vi "5RobotsFactorPass.vi"(0 "Utilities in":refnum<class "Utilities.lvclass">, 1 "ID":dbl, 5 "Game in":refnum<class "Game.lvclass">, 7 "reference":refnum<class "Enemy.lvclass">, 9 "Root":dbl=1.0, 11 "error in (no error)":errorcluster, 12 "Pass?":bool, 13 "Enemy?":bool, 14 "dest_kick":dbl[][](array[numeric])) -> (3 "Debug":dbl[][](array[numeric]), 4 "Utilities out":refnum<class "Utilities.lvclass">, 6 "Id":i32[](array[numeric]), 10 "FactorPass":dbl[](array[numeric]), 15 "error out":errorcluster)   [LabVIEW 2021, in "Utilities.lvclass"]
uses:
  Utilities.lvclass
  Game_class/Game.lvclass
  Enemy_class/Enemy.lvclass
  D:/RoboIme/horie/SSL_AI/Team_class/Team.lvclass
  Game_class/Game.lvclass/Game.ctl
  Team_class/Team.lvclass/Team.ctl
  Object_class/Object.lvclass/Object.ctl
  Robot_class/roles.ctl
  Robot_class/Robot.lvclass/Robot.ctl
  Team_class/OffensivePlay.ctl
  Referee_class/Referee.lvclass/Referee.ctl
  Object_class/Read position(x,y).vi
  Team_class/Read RobotRef.vi
  Robot_class/Read id.vi
  Object_class/Read x.vi
  Object_class/Read y.vi
  Referee_class/Read enemy_goalie_id.vi
  Referee_class/Read our_goalie_id.vi
  Game_class/Read OffensiveTeam.vi
  Game_class/Read BallRef.vi
  Game_class/Read FieldRef.vi
  Game_class/Read EnemyRef.vi
  Game_class/Read Referee.vi
  Ally_class/Ally.lvclass
  Robot_class/Robot.lvclass
  D:/RoboIme/horie/SSL_AI/Object_class/Object.lvclass
  Ball_class/Ball.lvclass
  Field_class/Field.lvclass
  Referee_class/Referee.lvclass
  Team_class/Team.lvclass
panel:
  in  "y3 2":dbl=0.2
  in  "y4 2":dbl=0.2
  in  "y":dbl=0.2
  in  "y2":dbl=0.22
  in  "y3":dbl=0.35
  in  "y4":dbl=0.16
  in  "y5":dbl=0.07
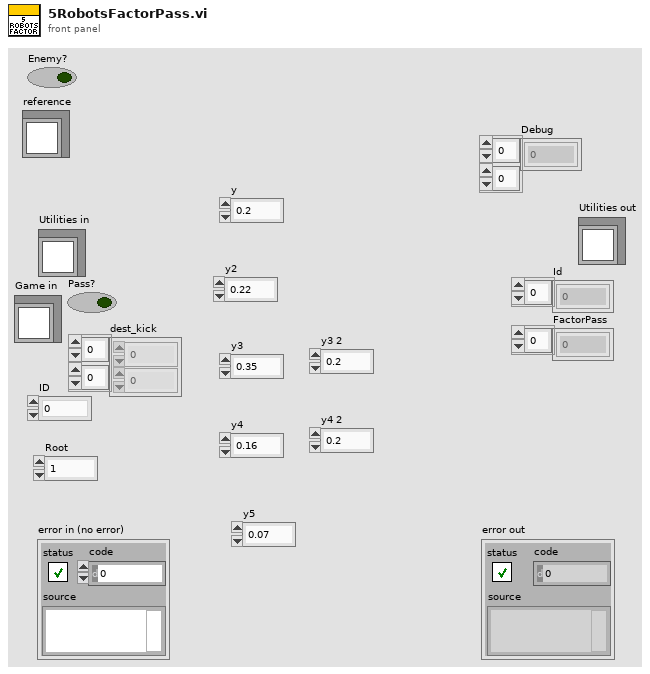
[diagram p1: front panel]
types:
  T1 = typedef "roles.ctl" = enum16{"SimpleBallPlacement", "BallPlacementAllyPasser", "BallPlacementAllyReceiver", "BallPlacementEnemy", "5Robots5th", "PassBestReceiver", "5Robots4th", "5Robots3rd", "5Robots2nd", "5Robots1st", "PassBestRobot", "WaitPass", "ABCThirdKicker", "ABCFirstKicker", "ABCSecondKicker", "Tabler", "TableFinalizer", "PrepareRollToPassRoller", "PrepareRollToPassReceiver", "SimplePassRoll", "SimplePassRollReceiver", "PenaltyDefense", "PreparePassReceiver 2", "PreparePassReceiver 1", "PassObserver", "Timeout", "Goto", "ZigZag", "None", "BallOutOfField", "DefenderArea", "Duelist", "AttackerStop", "FollowAttacker", "KeeperRole", "KickPenalty", "AttackerAimGoal", "AttackerBlock", "Marker", "Halt", "Shoot", "PassKicker", "PassReceiver", "TestRole", "PenaltyAttacker"}
  T2 = typedef "OffensivePlay.ctl" = enum16{"5RobotsPassGamePlay", "5PreparePassGame", "5RobotsKeeperGame", "KeeperPassToStriker", "5RobotsNormalGamePlay", "PrepareKeeperPass", "ACBPass", "ABCPass", "PrepareTriplePass", "TableWithStriker", "TableWith2ndStrikerPlay", "PrepareDoublePass", "PrepareRollToPass", "SimplePass", "PreparePass", "PassToStriker", "BallOutOfField", "PassTo2ndStriker", "StopOffensive", "Prepare Penalty Enemy", "EnemyPossessionAtEnemyField", "EnemyPossesionAtOurField", "TestPlay", "PreparePenaltyAlly", "KickPenaltyAlly", "PrepareKickoffAlly", "PrepareKickoffEnemy", "IndirectEnemy", "DirectEnemy", "PreparePassInGame1", "NormalGame", "DirectKick", "Pass", "Halt", "Timeout", "PassPlay", "PenaltyEnemy"}
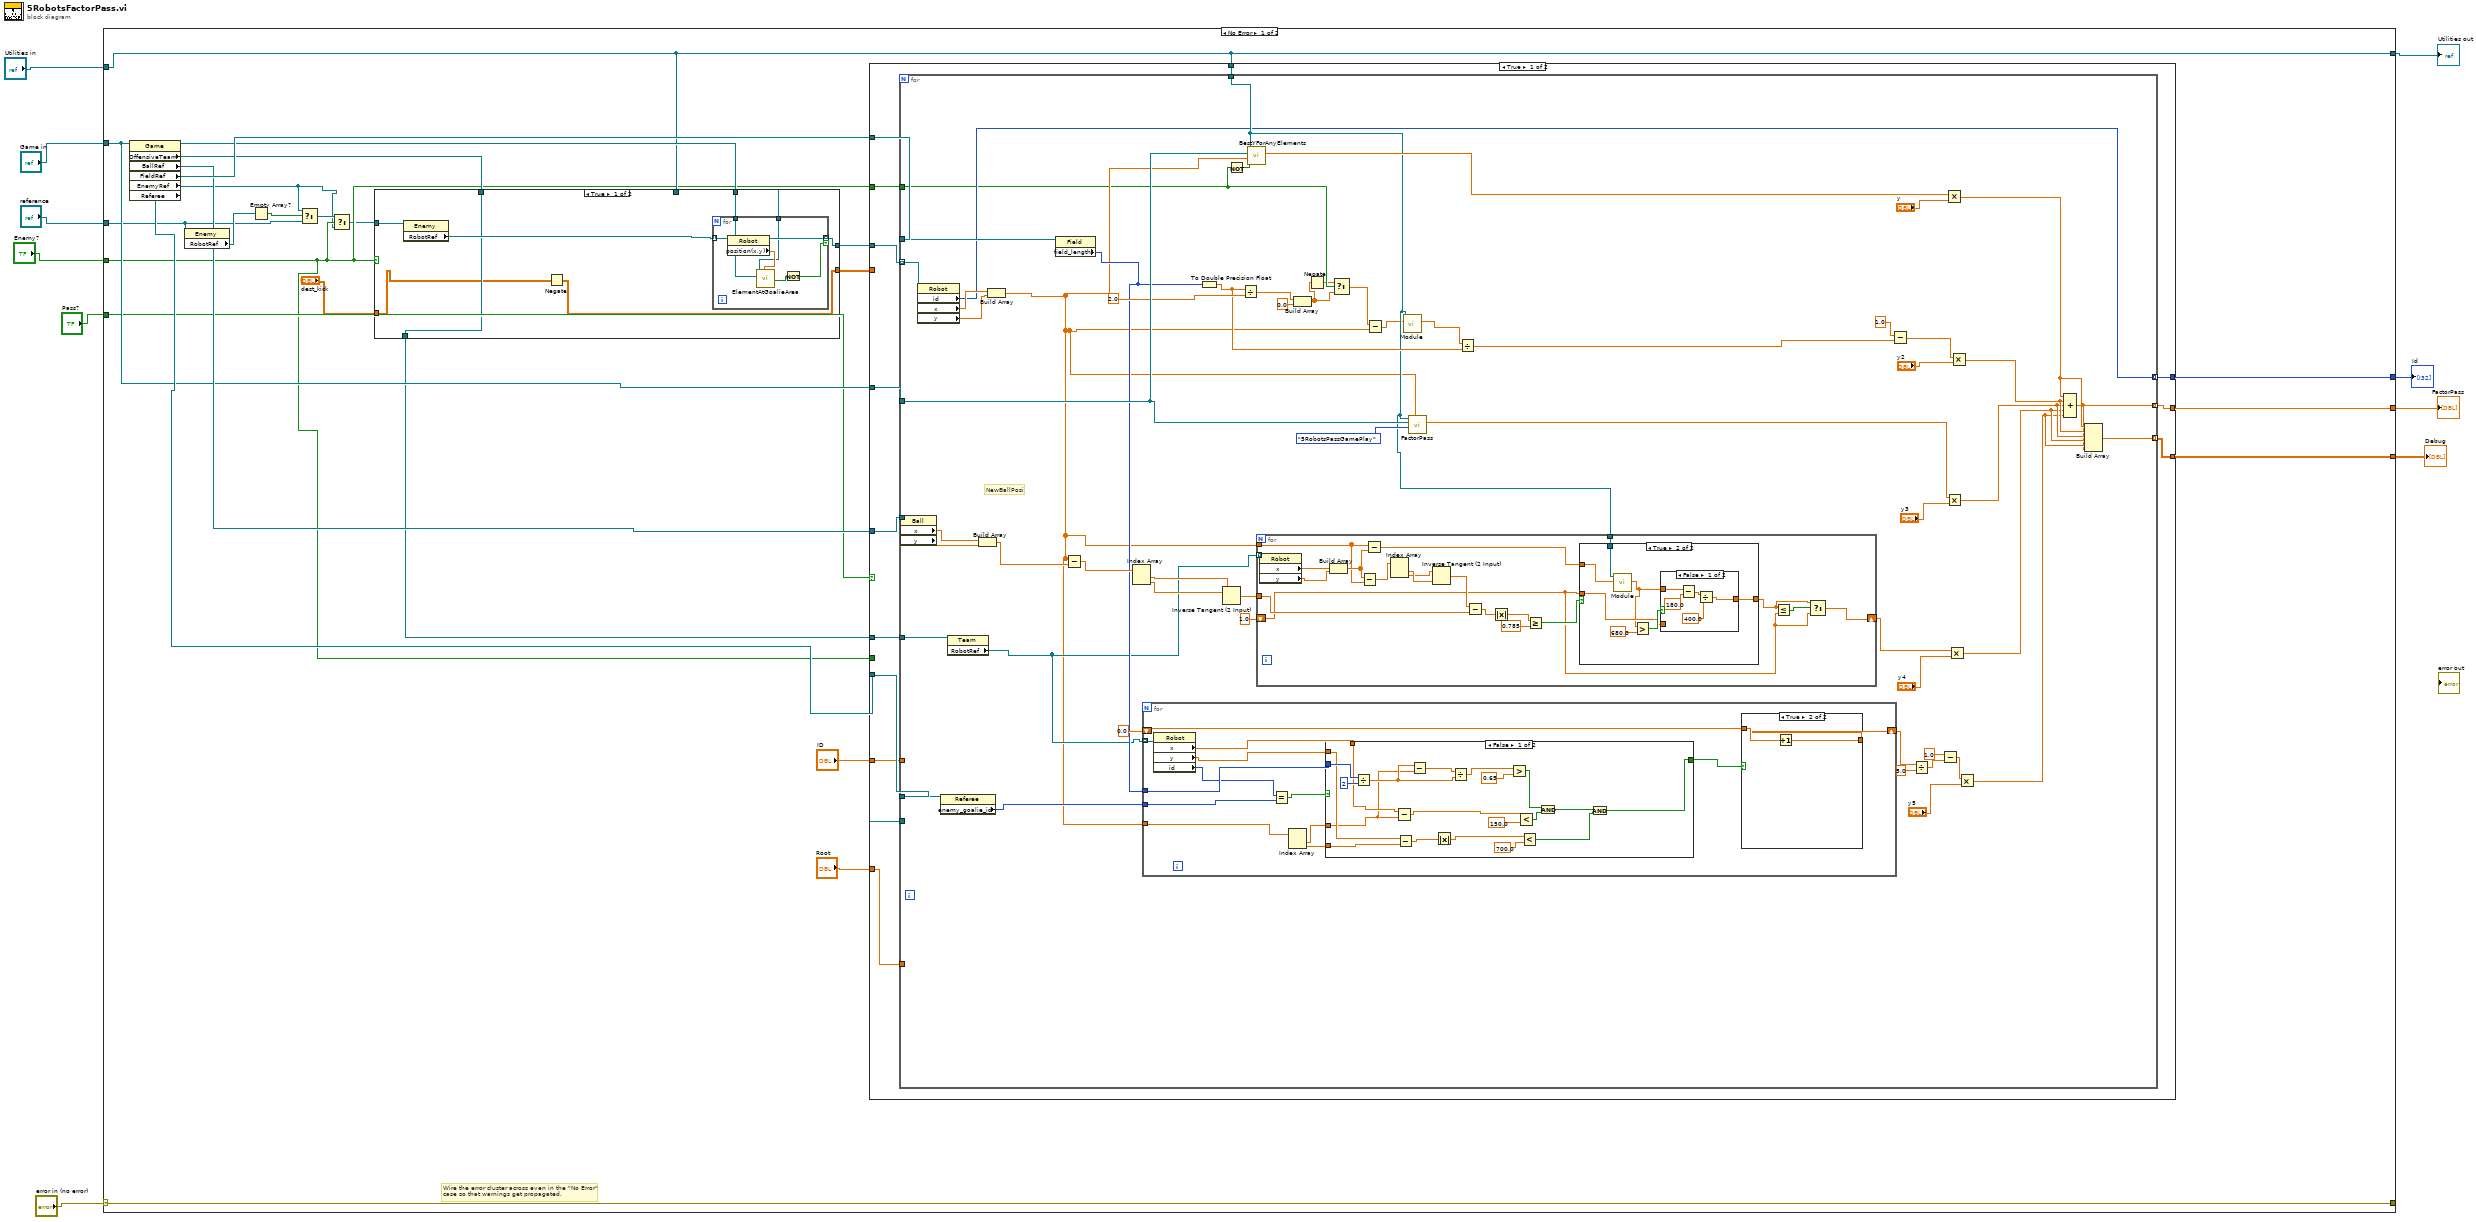
[diagram p0: block diagram]
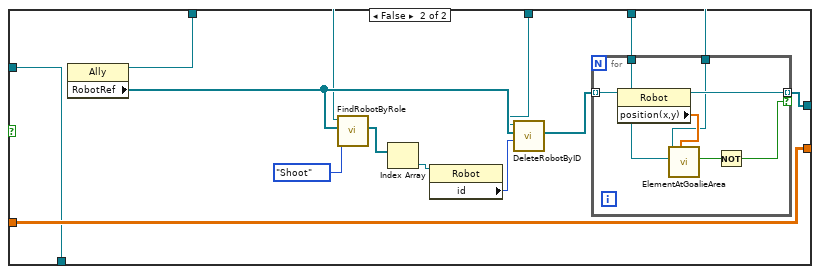
[diagram p2: hidden frame]
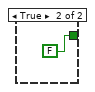
[diagram p3: hidden frame]
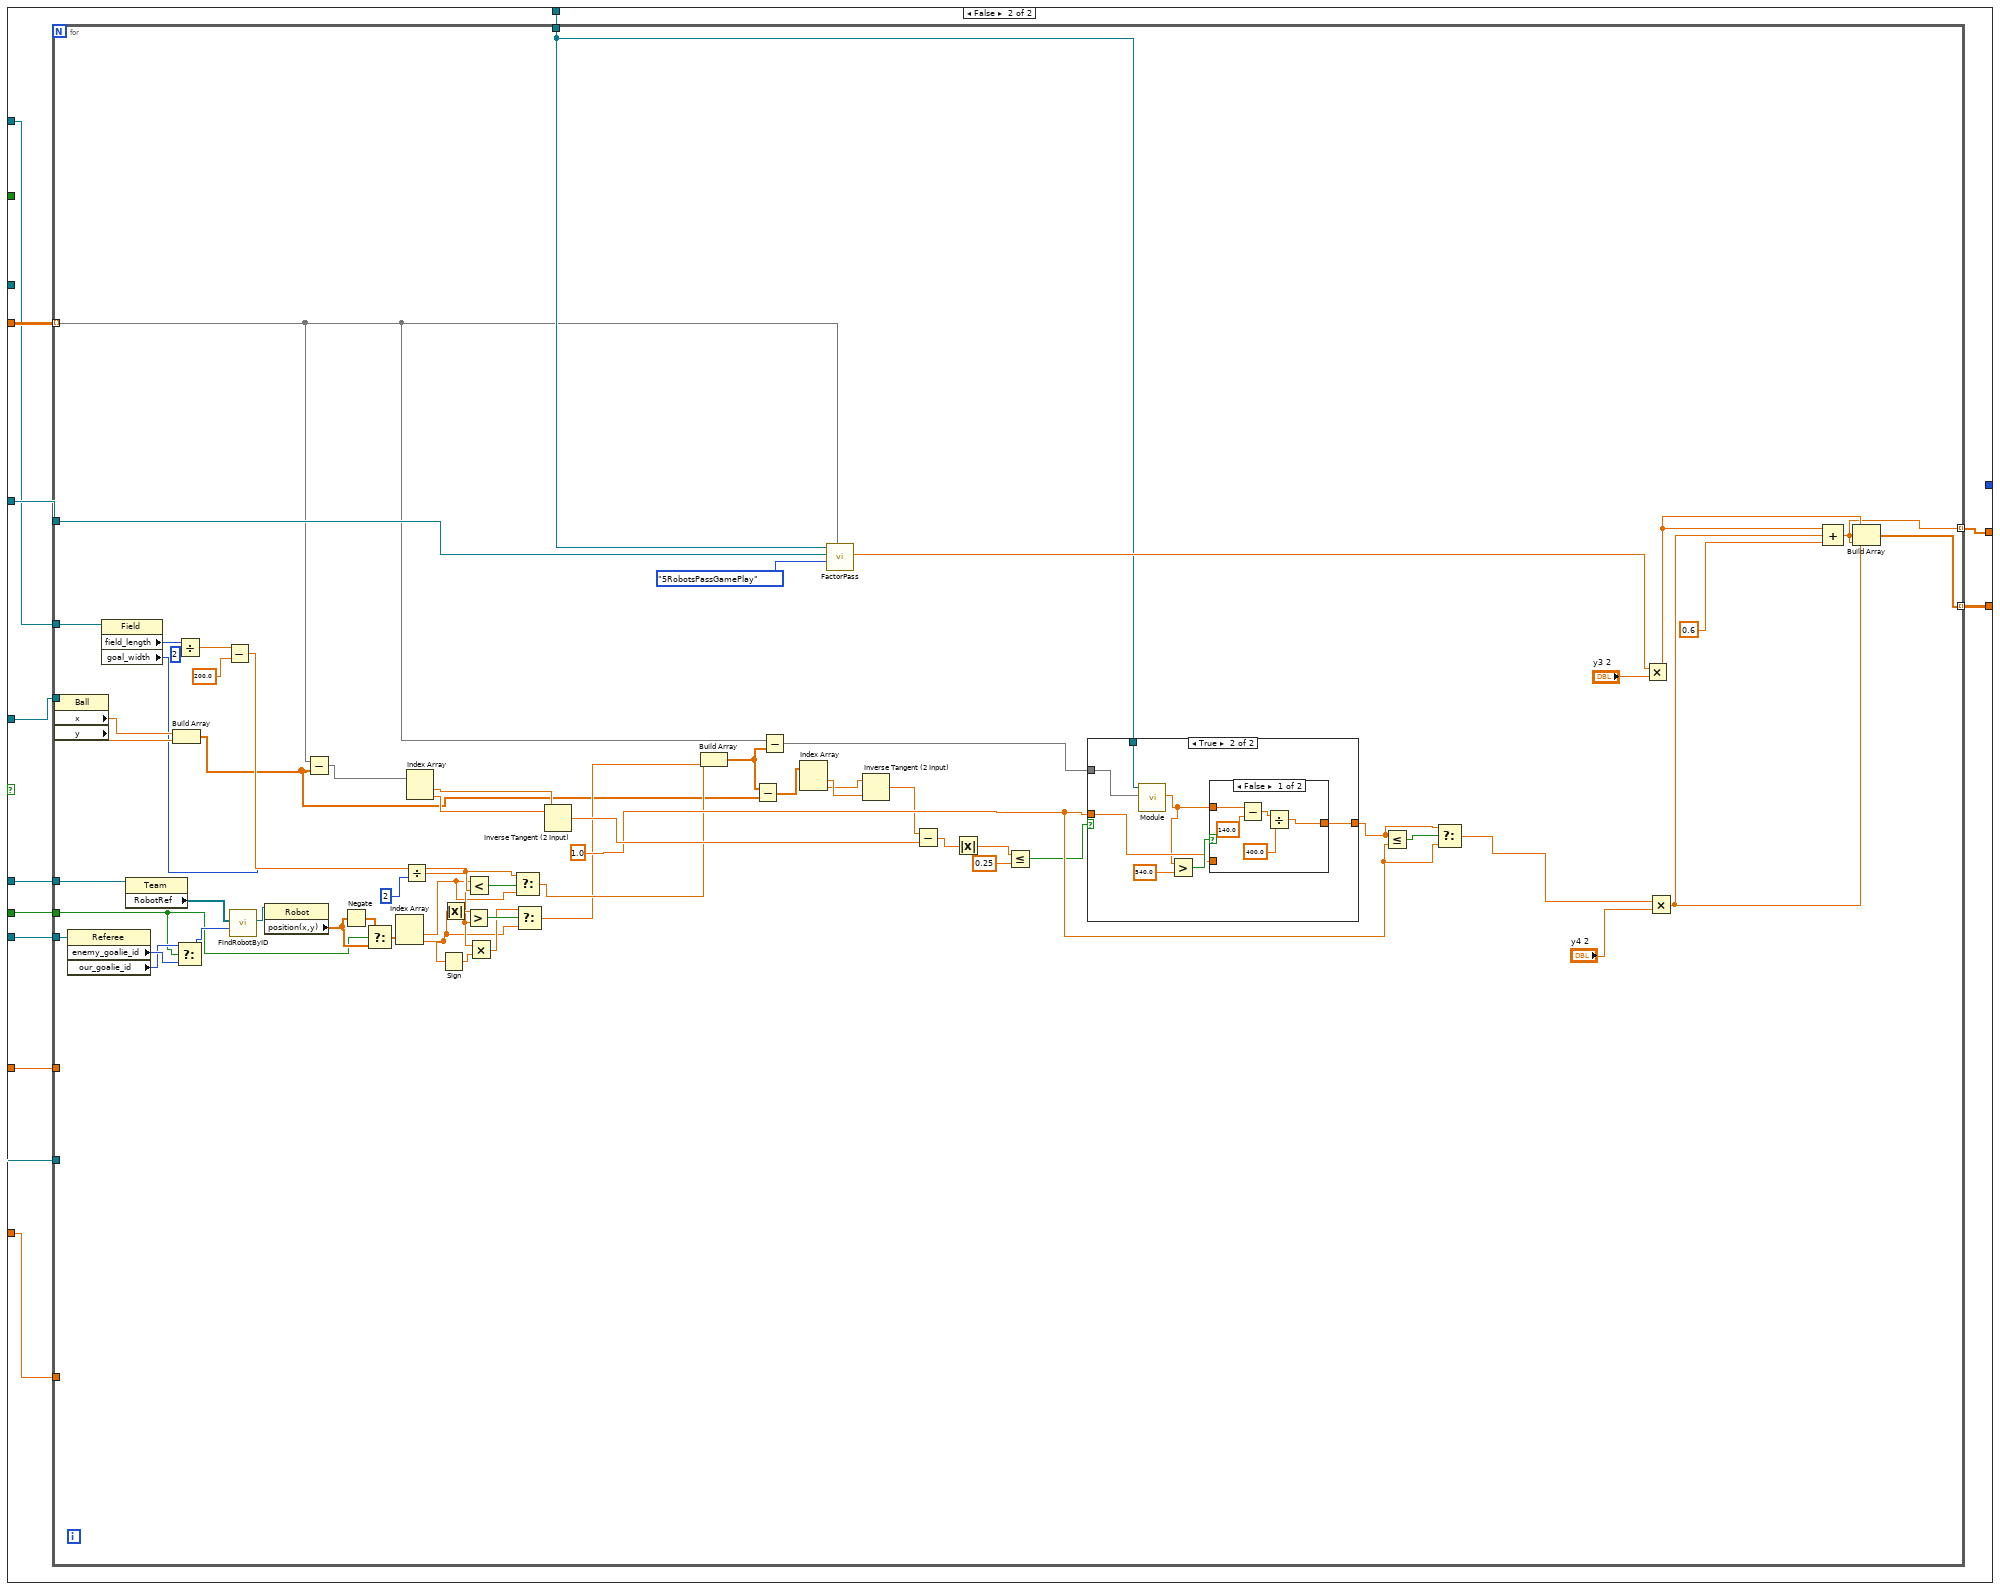
[diagram p7: hidden frame]
diagram:
  n1 = case shown="No Error" "error in (no error)" {
    selector: "error in (no error)" -> [w35 w302]
    tunnel: [w35 w302] -> _
    tunnel: [w31 _] -> w6
    tunnel: "Utilities in" -> [w20 w301]
    tunnel: [w20 w301] -> w10
    tunnel: "Game in" -> [w28 _]
    tunnel: [w29 _] -> w7
    tunnel: "Pass?" -> [w26 _]
    tunnel: [w24 _] -> w3
    tunnel: "Enemy?" -> [w14 _]
    tunnel: "reference" -> [w15 _]
    frame No Error {
      # "Wire the error cluster across even in the \"No Error\"\ncase so that warnings get propagated."
      n2 = property class="Game"(reference=w28) -> (reference out=w22:refnum<class "Game.lvclass">, "OffensiveTeam"=w30:refnum<class "Ally.lvclass">, "BallRef"=w33:refnum<class "Ball.lvclass">, "FieldRef"=w34:refnum<class "Field.lvclass">, "EnemyRef"=w11:refnum<class "Enemy.lvclass">, "Referee"=w32:refnum<class "Referee.lvclass">)  [unwired: 1 in, 1 out]
      n3 = property class="Enemy"(reference=w15) -> ("RobotRef"=w16:refnum<class "Robot.lvclass">[])  [unwired: 1 in, 2 out]
      n4 = Empty Array?(array=w16) -> (empty?=w17:bool)
      n5 = Select(t=w11, s=w17, f=w15) -> (s? t:f=w12:refnum<class "Enemy.lvclass">)
      n6 = Select(t=w12, s=w14, f=w11) -> (s? t:f=w13:refnum<class "Enemy.lvclass">)
      n7 = case shown="True" w14 {
        tunnel: w30 -> [w39 w62]
        tunnel: [w37 w52] -> w25
        tunnel: w22 -> [w43 w56]
        tunnel: [w42 w54] -> w21
        tunnel: w20 -> [w41 w53]
        tunnel: "dest_kick" -> [w38 w52]
        tunnel: [w39 w51] -> w18
        tunnel: w13 -> [w36 w51]
        frame True {
          n8 = property class="Enemy"(reference=w36) -> ("RobotRef"=w40:refnum<class "Robot.lvclass">[])  [unwired: 1 in, 2 out]
          n9 = Negate(x=w38) -> (-x=w37:dbl[][])
          n10 = for {
            tunnel: w43 -> [w50]
            tunnel: w40 -> [w49] mode=indexing
            tunnel: [w47] -> w42 mode=indexing if=w46
            tunnel: w41 -> [w45]
            n11 = property class="Robot"(reference=w49) -> (reference out=w47:refnum<class "Robot.lvclass">, "position(x,y)"=w48:dbl[])  [unwired: 1 in, 1 out]
            n12 = call "ElementAtGoalieArea.vi"("Elemento pos."=w48, "Game"=w50, "Utilities in"=w45) -> ("Element at our goalkeeper area ?"=w44:bool)  [unwired: 4 in, 4 out]
            n13 = Not(x=w44) -> (.not. x?=w46:bool)
          }
        }
        frame False {
          n14 = property class="Ally"(reference=w62) -> ("RobotRef"=w57:refnum<class "Robot.lvclass">[])  [unwired: 1 in, 2 out]
          n15 = call "FindRobotByRole.vi"("role"=roles."Shoot", "RobotRef"=w57, "Utilities in"=w53) -> ("Robots"=w60:refnum<class "Robot.lvclass">[])  [unwired: 6 in, 2 out]
          n16 = Index Array(array=w60) -> (element=w59:refnum<class "Robot.lvclass">)  [unwired: 1 in]
          n17 = property class="Robot"(reference=w59) -> ("id"=w58:i32)  [unwired: 1 in, 2 out]
          n18 = call "DeleteRobotByID.vi"("id"=w58, "RobotRef"=w57, "Utilities in"=w53) -> ("RobotRef out"=w55:refnum<class "Robot.lvclass">[])  [unwired: 6 in, 2 out]
          n19 = for {
            tunnel: w56 -> [w69]
            tunnel: w55 -> [w68] mode=indexing
            tunnel: [w66] -> w54 mode=indexing if=w64
            tunnel: w53 -> [w63]
            n20 = property class="Robot"(reference=w68) -> (reference out=w66:refnum<class "Robot.lvclass">, "position(x,y)"=w67:dbl[])  [unwired: 1 in, 1 out]
            n21 = call "ElementAtGoalieArea.vi"("Elemento pos."=w67, "Game"=w69, "Utilities in"=w63) -> ("Element at any goalkeeper area ?"=w65:bool)  [unwired: 4 in, 4 out]
            n22 = Not(x=w65) -> (.not. x?=w64:bool)
          }
        }
      }
      n23 = case shown="True" w26 {
        tunnel: w34 -> [w82 w213]
        tunnel: w33 -> [w81 w223]
        tunnel: w18 -> [w80 w222]
        tunnel: w32 -> [w79 w214]
        tunnel: [w78 w221] -> w31
        tunnel: w20 -> [w77 w220]
        tunnel: w21 -> [w76 _]
        tunnel: [w75 _] -> w29
        tunnel: w28 -> [w74 w219]
        tunnel: "ID" -> [w73 w218]
        tunnel: "Root" -> [w72 w215]
        tunnel: w25 -> [_ w217]
        tunnel: [w71 w216] -> w24
        tunnel: w14 -> [w70 _]
        tunnel: w14 -> [_ w212]
        frame True {
          n24 = for {
            tunnel: w82 -> [w140]
            tunnel: w81 -> [w139]
            tunnel: w80 -> [w138]
            tunnel: w79 -> [w137]
            tunnel: [w90] -> w78 mode=indexing
            tunnel: w74 -> [w136]
            tunnel: w77 -> [w100]
            tunnel: w76 -> [w104] mode=indexing
            tunnel: [w99] -> w75 mode=indexing
            tunnel: w72 -> [_]
            tunnel: w74 -> [_]
            tunnel: w73 -> [_]
            tunnel: [w93] -> w71 mode=indexing
            tunnel: w70 -> [w86]
            # "NewBallPosi"
            n25 = property class="Ball"(reference=w139) -> ("x"=w124:dbl, "y"=w123:dbl)  [unwired: 1 in, 2 out]
            n26 = property class="Robot"(reference=w104) -> ("id"=w99:i32, "x"=w103:dbl, "y"=w102:dbl)  [unwired: 1 in, 2 out]
            n27 = property class="Referee"(reference=w137) -> ("enemy_goalie_id"=w106:i32)  [unwired: 1 in, 2 out]
            n28 = property class="Team"(reference=w138) -> ("RobotRef"=w107:refnum<class "Robot.lvclass">[])  [unwired: 1 in, 2 out]
            n29 = Build Array(w124, w123) -> (w89:dbl[])
            n30 = Build Array(w103, w102) -> (w87:dbl[])
            n31 = property class="Field"(reference=w140) -> ("field_length"=w109:i32)  [unwired: 1 in, 2 out]
            n32 = Subtract(x=w87, y=w89) -> (x-y=w122:dbl[])
            n33 = Index Array(array=w122) -> (element #1=w120:dbl, element #2=w121:dbl)  [unwired: 2 in]
            n34 = for {
              tunnel: w87 -> [w147]
              shift-right: [w152] -> w115
              shift-left: 0.0 -> [w153]
              tunnel: w106 -> [w151]
              tunnel: w109 -> [w148]
              tunnel: w107 -> [w144] mode=indexing
              n35 = property class="Robot"(reference=w144) -> ("x"=w143:dbl, "y"=w142:dbl, "id"=w141:i32)  [unwired: 1 in, 2 out]
              n36 = Equal?(x=w141, y=w151) -> (x = y?=w150:bool)
              n37 = Index Array(array=w147) -> (element #1=w146:dbl, element #2=w145:dbl)  [unwired: 2 in]
              n38 = case shown="False" w150 {
                tunnel: [w155 FALSE] -> w149
                tunnel: w148 -> [w173 _]
                tunnel: w143 -> [w166 _]
                tunnel: w146 -> [w154 _]
                tunnel: w142 -> [w164 _]
                tunnel: w145 -> [w163 _]
                frame False {
                  n39 = Divide(x=w173, y=u32 2) -> (x/y=w170:dbl)
                  n40 = Subtract(x=w166, y=w154) -> (x-y=w165:dbl)
                  n41 = Subtract(x=w164, y=w163) -> (x-y=w162:dbl)
                  n42 = Subtract(x=w170, y=w154) -> (x-y=w171:dbl)
                  n43 = Absolute Value(x=w162) -> (abs(x)=w161:dbl)
                  n44 = Divide(x=w171, y=w170) -> (x/y=w169:dbl)
                  n45 = Greater?(x=w169, y=0.65) -> (0:w159:bool)
                  n46 = Less?(x=w165, y=150.0) -> (x < y?=w158:bool)
                  n47 = Less?(x=w161, y=700.0) -> (x < y?=w156:bool)
                  n48 = And(x=w159, y=w158) -> (x .and. y?=w157:bool)
                  n49 = And(x=w157, y=w156) -> (x .and. y?=w155:bool)
                }
                frame True {
                }
              }
              n50 = case shown="True" w149 {
                tunnel: w153 -> [w175 w177]
                tunnel: [w175 w176] -> w152
                frame False {
                }
                frame True {
                  n51 = Increment(x=w177) -> (x+1=w176:dbl)
                }
              }
            }
            n52 = To Double Precision Float(number=w109) -> (double precision float=w130:dbl)
            n53 = Inverse Tangent (2 Input)(1:w120, 2:w121) -> (0:w119:dbl)
            n54 = Not(x=w86) -> (.not. x?=w88:bool)
            n55 = Divide(x=w130, y=2.0) -> (x/y=w134:dbl)
            n56 = call "BestYForAnyElements.vi"("inimigos"=w88, "Position to be analyzed"=w87, "Game"=w136, "Utilities in"=w100) -> ("Goal Gap"=w108:dbl)  [unwired: 6 in, 1 out]
            n57 = for {
              tunnel: w119 -> [w192]
              tunnel: w87 -> [w182]
              shift-right: [w184] -> w118
              shift-left: 1.0 ("element") -> [w183]
              tunnel: w107 -> [w181] mode=indexing
              tunnel: w100 -> [w178]
              n58 = property class="Robot"(reference=w181) -> ("x"=w180:dbl, "y"=w179:dbl)  [unwired: 1 in, 2 out]
              n59 = Build Array(w180, w179) -> (w188:dbl[])
              n60 = Subtract(x=w188, y=w182) -> (x-y=w197:dbl[])
              n61 = Subtract(x=w182, y=w188) -> (x-y=w187:dbl[])
              n62 = Index Array(array=w197) -> (element #1=w194:dbl, element #2=w193:dbl)  [unwired: 2 in]
              n63 = Inverse Tangent (2 Input)(1:w194, 2:w193) -> (0:w196:dbl)
              n64 = Subtract(x=w196, y=w192) -> (x-y=w195:dbl)
              n65 = Absolute Value(x=w195) -> (abs(x)=w190:dbl)
              n66 = Greater Or Equal?(x=w190, y=0.785) -> (x >= y?=w189:bool)
              n67 = case shown="True" w189 {
                tunnel: w183 -> [w198 w202]
                tunnel: w187 -> [_ w201]
                tunnel: [w198 w204] -> w185
                tunnel: w178 -> [_ w200]
                frame False {
                }
                frame True {
                  n68 = call "Module.vi"("2D vector"=w201, "Utilities in"=w200) -> ("Modulo"=w199:dbl)  [unwired: 7 in, 2 out]
                  n69 = Greater?(x=w199, y=680.0) -> (0:w203:bool)
                  n70 = case shown="False" w203 {
                    tunnel: w202 -> [_ w211]
                    tunnel: [w210 w211] -> w204
                    tunnel: w199 -> [w206 _]
                    frame False {
                      n71 = Subtract(x=w206, y=180.0) -> (x-y=w208:dbl)
                      n72 = Divide(x=w208, y=400.0) -> (x/y=w210:dbl)
                    }
                    frame True {
                    }
                  }
                }
              }
              n73 = Less Or Equal?(x=w185, y=w183) -> (x <= y?=w186:bool)
              n74 = Select(t=w185, s=w186, f=w183) -> (s? t:f=w184:dbl)
            }
            n75 = Build Array(w134, 0.0 ("element")) -> (w85:dbl[])
            n76 = Negate(x=w85) -> (-x=w84:dbl[])
            n77 = Select(t=w84, s=w86, f=w85) -> (s? t:f=w83:dbl[])
            n78 = Subtract(x=w83, y=w87) -> (x-y=w92:dbl[])
            n79 = call "Module.vi"("2D vector"=w92, "Utilities in"=w100) -> ("Modulo"=w91:dbl)  [unwired: 7 in, 2 out]
            n80 = call-dynamic "FactorPass.vi"("Robot"=w87, "OffensivePlay"=OffensivePlay."5RobotsPassGamePlay", "Game"=w136, "Utilities in"=w100) -> ("Critério de marcação Normalizado"=w105:dbl)  [unwired: 5 in, 2 out]
            n81 = Divide(x=w91, y=w130) -> (x/y=w132:dbl)
            n82 = Subtract(x=1.0, y=w132) -> (x-y=w129:dbl)
            n83 = Divide(x=w115, y=5.0) -> (x/y=w113:dbl)
            n84 = Subtract(x=1.0, y=w113) -> (x-y=w111:dbl)
            n85 = Multiply(x=w108, y="y") -> (x*y=w98:dbl)
            n86 = Multiply(x=w105, y="y3") -> (x*y=w96:dbl)
            n87 = Multiply(x=w118, y="y4") -> (x*y=w95:dbl)
            n88 = Multiply(x=w129, y="y2") -> (x*y=w97:dbl)
            n89 = Multiply(x=w111, y="y5") -> (x*y=w94:dbl)
            n90 = Compound Arithmetic op=ADD(w98, w97, w96, w95, w94) -> (w90:dbl)
            n91 = Build Array(w98, w97, w96, w95, w94, w90) -> (w93:dbl[])
          }
        }
        frame False {
          n92 = for {
            tunnel: w223 -> [w286]
            tunnel: w222 -> [w285]
            tunnel: [w267] -> w221 mode=indexing
            tunnel: w219 -> [w284]
            tunnel: w220 -> [w271]
            tunnel: w215 -> [_]
            tunnel: w219 -> [_]
            tunnel: w218 -> [_]
            tunnel: w217 -> [w224] mode=indexing
            tunnel: [w270] -> w216 mode=indexing
            tunnel: w214 -> [w264]
            tunnel: w213 -> [w263]
            tunnel: w212 -> [w228]
            w274 = 1.0 ("element")
            n93 = property class="Ball"(reference=w286) -> ("x"=w281:dbl, "y"=w280:dbl)  [unwired: 1 in, 2 out]
            n94 = property class="Referee"(reference=w264) -> ("enemy_goalie_id"=w232:i32, "our_goalie_id"=w231:i32)  [unwired: 1 in, 2 out]
            n95 = property class="Field"(reference=w263) -> ("field_length"=w262:i32, "goal_width"=w254:i32)  [unwired: 1 in, 2 out]
            n96 = property class="Team"(reference=w285) -> ("RobotRef"=w265:refnum<class "Robot.lvclass">[])  [unwired: 1 in, 2 out]
            n97 = Build Array(w281, w280) -> (w234:dbl[])
            n98 = Select(t=w231, s=w228, f=w232) -> (s? t:f=w233:i32)
            n99 = Divide(x=w262, y=2) -> (x/y=w260:dbl)
            n100 = Subtract(x=w260, y=200.0) -> (x-y=w256:dbl)
            n101 = call "FindRobotByID.vi"("id"=w233, "RobotRef"=w265) -> ("Robot"=w258:refnum<class "Robot.lvclass">)  [unwired: 6 in, 3 out]
            n102 = property class="Robot"(reference=w258) -> ("position(x,y)"=w230:dbl[])  [unwired: 1 in, 2 out]
            n103 = Subtract(x=w224, y=w234) -> (x-y=w279:dbl[])
            n104 = Negate(x=w230) -> (-x=w229:dbl[])
            n105 = Select(t=w229, s=w228, f=w230) -> (s? t:f=w227:dbl[])
            n106 = Index Array(array=w227) -> (element #1=w226:dbl, element #2=w225:dbl)  [unwired: 2 in]
            n107 = Divide(x=w254, y=2) -> (x/y=w250:dbl)
            n108 = Index Array(array=w279) -> (element #1=w277:dbl, element #2=w278:dbl)  [unwired: 2 in]
            n109 = Sign(1:w225) -> (0:w249:dbl)
            n110 = Absolute Value(x=w225) -> (abs(x)=w252:dbl)
            n111 = Greater?(x=w252, y=w250) -> (0:w251:bool)
            n112 = Less?(x=w226, y=w256) -> (x < y?=w257:bool)
            n113 = Multiply(x=w250, y=w249) -> (x*y=w248:dbl)
            n114 = Select(t=w256, s=w257, f=w226) -> (s? t:f=w255:dbl)
            n115 = Select(t=w248, s=w251, f=w225) -> (s? t:f=w247:dbl)
            n116 = Inverse Tangent (2 Input)(1:w277, 2:w278) -> (0:w276:dbl)
            n117 = Build Array(w255, w247) -> (w235:dbl[])
            n118 = Subtract(x=w235, y=w234) -> (x-y=w246:dbl[])
            n119 = Subtract(x=w224, y=w235) -> (x-y=w238:dbl[])
            n120 = Index Array(array=w246) -> (element #1=w243:dbl, element #2=w242:dbl)  [unwired: 2 in]
            n121 = call-dynamic "FactorPass.vi"("Robot"=w224, "OffensivePlay"=OffensivePlay."5RobotsPassGamePlay", "Game"=w284, "Utilities in"=w271) -> ("Critério de marcação Normalizado"=w273:dbl)  [unwired: 5 in, 2 out]
            n122 = Inverse Tangent (2 Input)(1:w243, 2:w242) -> (0:w245:dbl)
            n123 = Subtract(x=w245, y=w276) -> (x-y=w244:dbl)
            n124 = Absolute Value(x=w244) -> (abs(x)=w240:dbl)
            n125 = Less Or Equal?(x=w240, y=0.25) -> (x <= y?=w239:bool)
            n126 = case shown="True" w239 {
              tunnel: w274 -> [w287 w291]
              tunnel: w238 -> [_ w290]
              tunnel: [w287 w293] -> w236
              tunnel: w271 -> [_ w289]
              frame False {
              }
              frame True {
                n127 = call "Module.vi"("2D vector"=w290, "Utilities in"=w289) -> ("Modulo"=w288:dbl)  [unwired: 7 in, 2 out]
                n128 = Greater?(x=w288, y=540.0) -> (0:w292:bool)
                n129 = case shown="False" w292 {
                  tunnel: w291 -> [_ w300]
                  tunnel: [w299 w300] -> w293
                  tunnel: w288 -> [w295 _]
                  frame False {
                    n130 = Subtract(x=w295, y=140.0) -> (x-y=w297:dbl)
                    n131 = Divide(x=w297, y=400.0) -> (x/y=w299:dbl)
                  }
                  frame True {
                  }
                }
              }
            }
            n132 = Less Or Equal?(x=w236, y=w274) -> (x <= y?=w237:bool)
            n133 = Select(t=w236, s=w237, f=w274) -> (s? t:f=w275:dbl)
            n134 = Multiply(x=w273, y="y3 2") -> (x*y=w269:dbl)
            n135 = Multiply(x=w275, y="y4 2") -> (x*y=w268:dbl)
            n136 = Compound Arithmetic op=ADD(w269, w268, 0.6 ("element")) -> (w267:dbl)
            n137 = Build Array(w269, w268, w267) -> (w270:dbl[])
          }
        }
      }
    }
    frame Error {
    }
  }
  "Utilities out" <- w10
  "Id" <- w7
  "FactorPass" <- w6
  "Debug" <- w3
